vi "string to channel.vi"(10 "channel data":string, 11 "identifier":string) -> (3 "channel in":refnum<class "TBM channel.lvclass">)   [LabVIEW 2013, in "TBM channel.lvclass"]
uses:
  TBM channel.lvclass
  <vilib>/NI/Tag Bus/tag/Data Type.ctl
  channel classification.ctl
  <vilib>/NI/Tag Bus/tag/tag descriptor.lvclass/tag descriptor.ctl
  root configuration/TBM configuration.lvclass
  <vilib>/NI/Tag Bus/tag/tag descriptor.lvclass
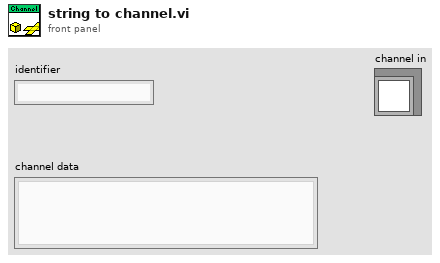
[diagram p1: front panel]
types:
  T1 = typedef "TBM channel.lvclass/channel classification.ctl" = enum16{"input data", "output data", "processing parameter", "processing result"}
  T2 = typedef "tag bus.lvlib/tag descriptor.lvclass/Data Type.ctl" = enum16{"Double", "Single", "I64", "I32", "I16", "I8", "U64", "U32", "U16", "U8", "Boolean", "String", "Array of Double", "Array of Single", "Array of I64", "Array of I32", "Array of I16", "Array of I8", "Array of U64", "Array of U32", "Array of U16", "Array of U8", "Array of Boolean", "Array of String"}
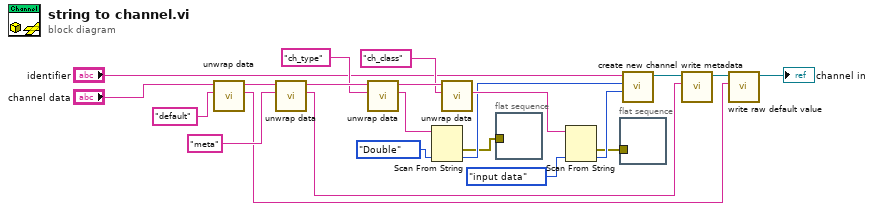
[diagram p0: block diagram]
diagram:
  n1 = call "unwrap data.vi"("identifier"="default", "data to unwrap"="channel data") -> ("unwrapped data"=w12:string, "remaining string"=w22:string)  [unwired: 8 in]
  n2 = call "unwrap data.vi"("identifier"="meta", "data to unwrap"=w22) -> ("unwrapped data"=w13:string, "remaining string"=w18:string)  [unwired: 8 in]
  n3 = call "unwrap data.vi"("identifier"="ch_type", "data to unwrap"=w18) -> ("unwrapped data"=w11:string, "remaining string"=w19:string)  [unwired: 8 in]
  n4 = Scan From String(input string=w11, default 1=Data_Type."Double" ("data type")) -> (error out=w5:errorcluster, output 1=w8:T2)  [unwired: 3 in, 2 out]
  n5 = call "unwrap data.vi"("identifier"="ch_class", "data to unwrap"=w19) -> ("unwrapped data"=w9:string)  [unwired: 8 in, 1 out]
  n6 = flat-sequence {
    tunnel: w5 -> [_]
    frame #0 {
    }
  }
  n7 = Scan From String(input string=w9, default 1=channel_classification."input data" ("channel classification")) -> (error out=w4:errorcluster, output 1=w6:T1)  [unwired: 3 in, 2 out]
  n8 = flat-sequence {
    tunnel: w4 -> [_]
    frame #0 {
    }
  }
  n9 = call "create new channel.vi"("channel classification"=w6, "data type"=w8, "channel name"="identifier") -> ("channel"=w15:refnum<class "TBM channel.lvclass">)  [unwired: 8 in]
  n10 = call <vilib>:"write metadata.vi"("metadata"=w13, "system tag in"=w15) -> ("system tag out"=w14:refnum<class "TBM channel.lvclass">)  [unwired: 8 in, 1 out]
  n11 = call <vilib>:"write raw default value.vi"("raw default"=w12, "system tag in"=w14) -> ("system tag out"=→"channel in":refnum<class "TBM channel.lvclass">)  [unwired: 8 in, 1 out]
